vi "clickableRange.vi"(9 "Horizontal":i32, 10 "Left":i32, 11 "Width":u32) -> ()   [LabVIEW 2020]
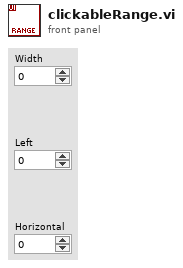
[diagram p1: front panel]
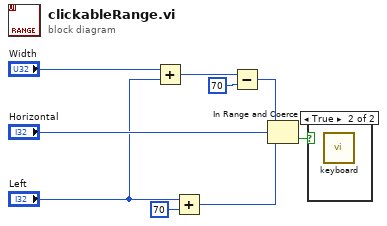
[diagram p0: block diagram]
diagram:
  n1 = Add(x="Width", y="Left") -> (x+y=w7:u32)
  n2 = Add(x="Left", y=70 ("x")) -> (x+y=w2:i32)
  n3 = Subtract(x=w7, y=u32 70) -> (x-y=w1:u32)
  n4 = In Range and Coerce(upper limit=w1, x="Horizontal", lower limit=w2) -> (In Range?=w3:bool)  [unwired: 1 out]
  n5 = case shown="True" w3 {
    frame False {
    }
    frame True {
      n6 = call "keyboard.vi"() -> ()  [unwired: 12 in]
    }
  }
